vi "log end of saving images.vi"(8 "error in (no error)":errorcluster, 11 "Save Image in":refnum<class "Save Image.lvclass">) -> (0 "error out":errorcluster, 3 "Save Image out":refnum<class "Save Image.lvclass">)   [LabVIEW 2018, in "Save Image.lvclass"]
uses:
  Save Image.lvclass
  Save Image.lvclass/Save Image.ctl
  Channel/Channel.lvclass
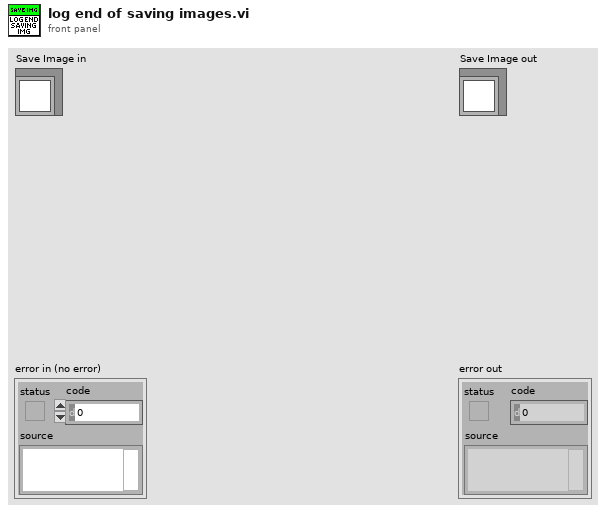
[diagram p1: front panel]
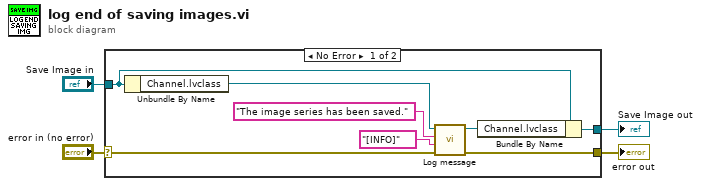
[diagram p0: block diagram]
diagram:
  n1 = case shown="No Error" "error in (no error)" {
    selector: "error in (no error)" -> [w7 w14]
    tunnel: [w8 w14] -> w3
    tunnel: [w11 w13] -> w1
    tunnel: "Save Image in" -> [w12 w13]
    frame No Error {
      n2 = Unbundle By Name(w12) -> ("Channel.lvclass"=w10:refnum<class "Channel.lvclass">)
      n3 = call "Log message.vi"("error in (no error)"=w7, "message type"="[INFO]", "String"="The image series has been saved.", "Channel in"=w10) -> ("error out"=w8:errorcluster, "Channel out"=w9:refnum<class "Channel.lvclass">)  [unwired: 6 in]
      n4 = Bundle By Name(cluster=w12, "Channel.lvclass"=w9) -> (w11:refnum<class "Save Image.lvclass">)
    }
    frame Error {
    }
  }
  "error out" <- w3
  "Save Image out" <- w1
